vi "get ring control values.vi"(8 "error in (no error)":errorcluster, 11 "Ring Ref":refnum<vi>[](array[refnum])) -> (0 "error out":errorcluster, 2 "items":string[](array[string]))   [LabVIEW 2024, in "Ring Control Management.lvlib"]
doc: "This VI retrieves the current item names and their indexes (Value) from the controls referenced in the <b>Ring Ref</b> array and stores them in the <b>items</b> array.\n\nThe <b>items</b> array is structured as follows: name1, index1, name2, index2, and so on."
uses:
  Ring Control Management.lvlib
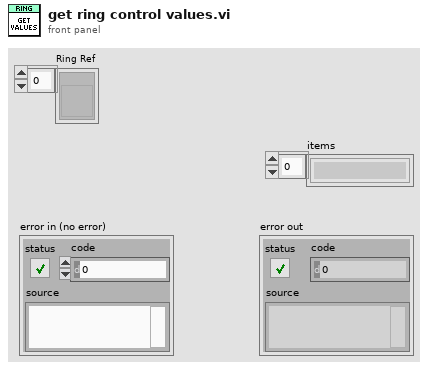
[diagram p1: front panel]
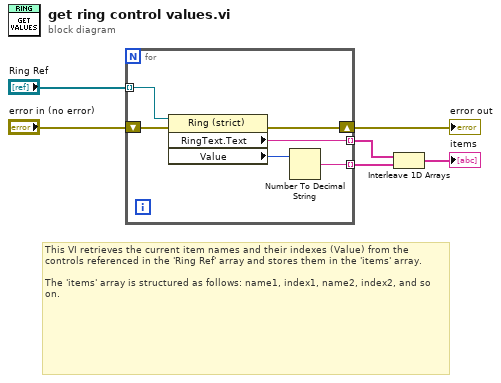
[diagram p0: block diagram]
diagram:
  # "This VI retrieves the current item names and their indexes (Value) from the controls referenced in the 'Ring Ref' array and stores them in the 'items' array.\n\nThe 'items' array is structured as follows: name1, index1, name2, index2, and so on."
  n1 = for {
    tunnel: "Ring Ref" -> [w11] mode=indexing
    tunnel: [w9] -> w1 mode=indexing
    tunnel: [w8] -> w2 mode=indexing
    shift-right: [w12] -> w6
    shift-left: "error in (no error)" -> [w7]
    n2 = property on="Property Node" class="Ring (strict)"(reference=w11, error in=w7) -> (error out=w12:errorcluster, "RingText.Text"=w9:string, "Value"=w10:u16)  [unwired: 1 out]
    n3 = Number To Decimal String(number=w10) -> (decimal integer string=w8:string)  [unwired: 1 in]
  }
  "error out" <- w6
  n4 = Interleave 1D Arrays(w1, w2) -> (→"items":string[])
